vi "Create Build Directory.vi"(8 "error in":errorcluster, 11 "base path":path) -> (0 "error out":errorcluster, 3 "build path":path)   [LabVIEW 2014]
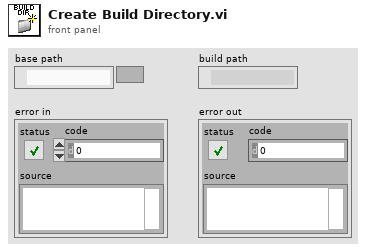
[diagram p1: front panel]
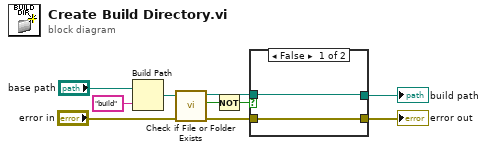
[diagram p0: block diagram]
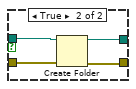
[diagram p2: hidden frame]
diagram:
  n1 = Build Path(base path="base path", name or relative path="build") -> (appended path=w3:path)
  n2 = call <vilib>:"Check if File or Folder Exists.vi"("error in (no error)"="error in", "path"=w3) -> ("error out"=w5:errorcluster, "file or folder exists?"=w6:bool, "dup path"=w10:path)  [unwired: 7 in]
  n3 = Not(x=w6) -> (.not. x?=w7:bool)
  n4 = case shown="False" w7 {
    tunnel: [w11 w15] -> w4
    tunnel: w5 -> [w11 w16]
    tunnel: [w12 w14] -> w9
    tunnel: w10 -> [w12 w13]
    frame False {
    }
    frame True {
      n5 = Create Folder(path (use dialog)=w13, error in=w16) -> (created path=w14:path, error out=w15:errorcluster)  [unwired: 1 in, 1 out]
    }
  }
  "build path" <- w9
  "error out" <- w4
